vi "enqueueMessage.vi"(7 "High Priority (F)":bool, 8 "error in (no error)":errorcluster, 11 "element":T1) -> (0 "error out":errorcluster)   [LabVIEW 2017, in "programControl.lvlib"]
uses:
  programControl.lvlib
  TypeDefs/message.ctl
  TypeDefs/queueFGVState.ctl
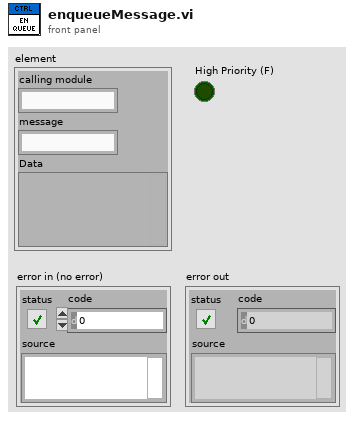
[diagram p1: front panel]
types:
  T1 = typedef "programControl.lvlib/message.ctl" = cluster{"calling module":string, "message":string, "Data":variant}
  T2 = typedef "programControl.lvlib/queueFGVState.ctl" = enum16{"get", "set"}
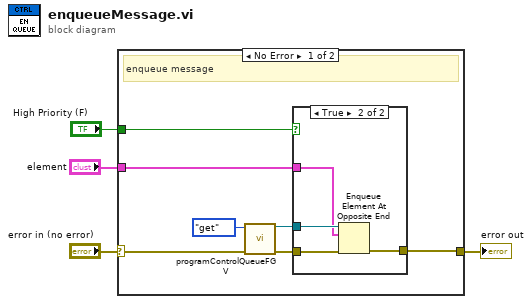
[diagram p0: block diagram]
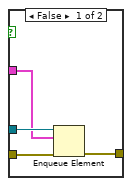
[diagram p2: hidden frame]
diagram:
  n1 = case shown="No Error" "error in (no error)" {
    selector: "error in (no error)" -> [w10 w20]
    tunnel: [w8 w20] -> w3
    tunnel: "element" -> [w6 _]
    tunnel: "High Priority (F)" -> [w5 _]
    frame No Error {
      # "enqueue message"
      n2 = call "programControlQueueFGV.vi"("error in (no error)"=w10, 11:queueFGVState."get") -> ("error out"=w9:errorcluster, "queue out"=w7:refnum<queue>)  [unwired: 8 in]
      n3 = case shown="True" w5 {
        tunnel: w9 -> [w15 w18]
        tunnel: [w14 w17] -> w8
        tunnel: w7 -> [w13 w19]
        tunnel: w6 -> [w12 w16]
        frame False {
          n4 = Enqueue Element(queue=w13, element=w12, error in (no error)=w15) -> (error out=w14:errorcluster)  [unwired: 1 in, 2 out]
        }
        frame True {
          n5 = Enqueue Element At Opposite End(queue=w19, element=w16, error in (no error)=w18) -> (error out=w17:errorcluster)  [unwired: 1 in, 2 out]
        }
      }
    }
    frame Error {
    }
  }
  "error out" <- w3
